vi "Write Tree Item Open State.vi"(8 "error in (no error)":errorcluster, 11 "File Explorer in":refnum<class "File Explorer.lvclass">) -> (0 "error out":errorcluster, 3 "File Explorer out":refnum<class "File Explorer.lvclass">)   [LabVIEW 2017, in "File Explorer.lvlib" / "File Explorer.lvclass"]
uses:
  <vilib>/gpm_packages/@cs/file-explorer-extension/Source/File Explorer/File Explorer/File Explorer.lvclass
  <vilib>/gpm_packages/@cs/file-explorer-extension/Source/File Explorer/File Explorer/File Explorer.lvclass/File Explorer.ctl
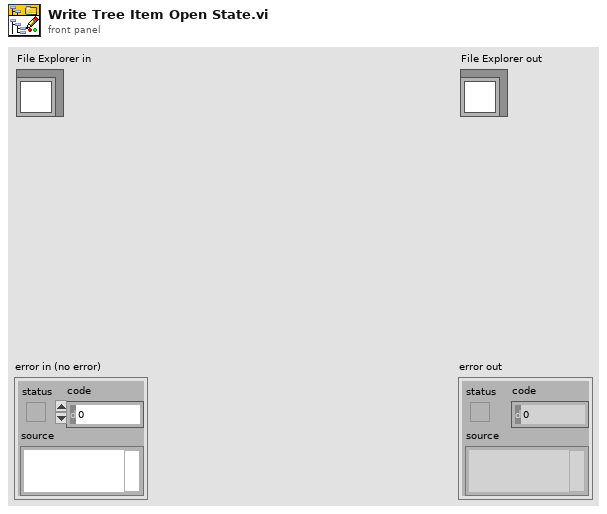
[diagram p1: front panel]
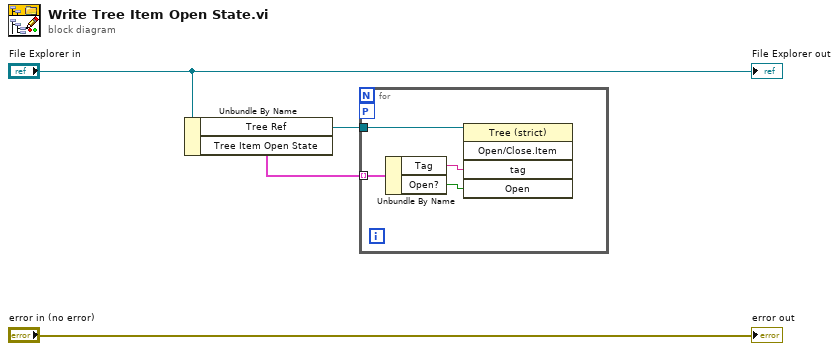
[diagram p0: block diagram]
diagram:
  n1 = Unbundle By Name("File Explorer in") -> ("Tree Ref"=w3:refnum<vi>, "Tree Item Open State"=w2:cluster{"Tag":string, "Open?":bool}[])
  n2 = for {
    tunnel: w2 -> [w7] mode=indexing
    tunnel: w3 -> [w8]
    workers-P: _ -> [_]
    n3 = Unbundle By Name(w7) -> ("Tag"=w6:string, "Open?"=w5:bool)
    n4 = invoke class="Tree (strict)" method="Open/Close.Item"(reference=w8, "tag"=w6, "Open"=w5) -> ()  [unwired: 2 in, 5 out]
  }
  "error out" <- "error in (no error)"
  "File Explorer out" <- "File Explorer in"
